vi "Spectrometer GetControlPosition.vi"(8 "error in":errorcluster, 9 "Control Refnum":refnum<vi>, 10 "Motor Name":T1=enum."Hole", 11 "Automation Refnum In":refnum<k7>) -> (0 "error out":errorcluster, 2 "Position":variant, 3 "Automation Refnum Out":refnum<k7>)   [LabVIEW 2014]
uses:
  MoveMotor Motor Name.ctl
  GetMotorPosition Mode.ctl
  Acquire Mode.ctl
panel:
  # "LICENSED MATERIALS – PROPERTY OF IBM\nCopyright IBM Corp. 2016,\nALL RIGHTS RESERVED"
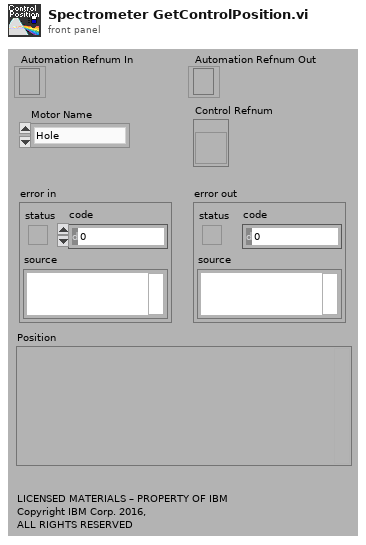
[diagram p1: front panel]
types:
  T1 = typedef "MoveMotor Motor Name.ctl" = enum16{"Spectro", "Premono", "Grating", "Slit", "Hole", "X", "Y", "XT", "YT", "XL", "YL", "Z", "Laser", "Filter", "Objective", "Detector", "Detector Temperature"}
  T2 = typedef "GetMotorPosition Mode.ctl" = u16
  T3 = typedef "Acquire Mode.ctl" = u16
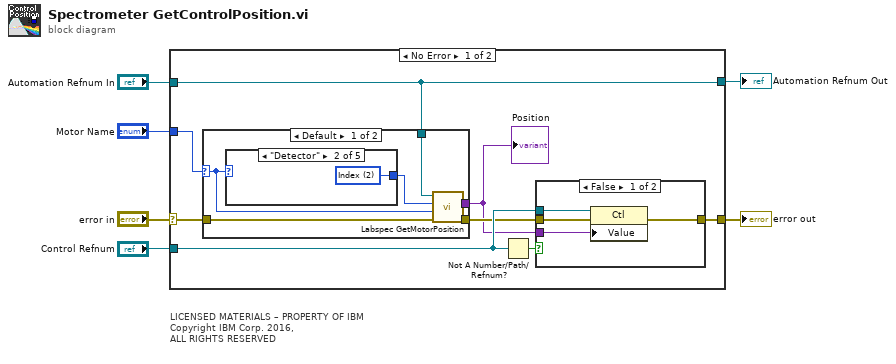
[diagram p0: block diagram]
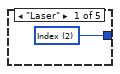
[diagram p2: hidden frame]
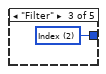
[diagram p3: hidden frame]
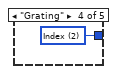
[diagram p4: hidden frame]
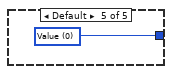
[diagram p5: hidden frame]
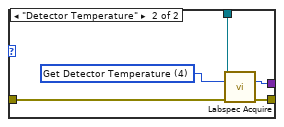
[diagram p6: hidden frame]
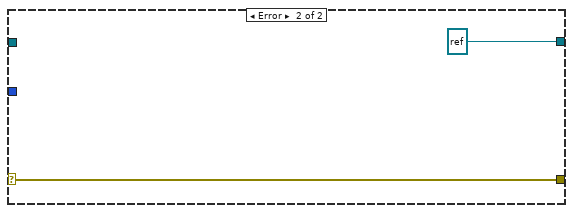
[diagram p8: hidden frame]
diagram:
  # "LICENSED MATERIALS – PROPERTY OF IBM\nCopyright IBM Corp. 2016,\nALL RIGHTS RESERVED"
  n1 = case shown="No Error" "error in" {
    selector: "error in" -> [w12 w37]
    tunnel: "Automation Refnum In" -> [w11 _]
    tunnel: [w11 refnum<k7> refnum ("Automation Refnum")] -> w5
    tunnel: "Motor Name" -> [w7 _]
    tunnel: [w13 w37] -> w3
    tunnel: "Control Refnum" -> [w14 _]
    frame No Error {
      n2 = case shown="Default" w7 {
        selector: w7 -> [w15 _]
        tunnel: w12 -> [w20 w27]
        tunnel: w11 -> [w19 w26]
        tunnel: [w18 w28] -> w10
        tunnel: [w17 w29] -> w9
        frame Default {
          n3 = case shown="\"Detector\"" w15 {
            tunnel: [w21 w22 w23 w24 w25] -> w16
            frame "Laser" {
              w21 = T2 2 items=["Value", "Step", "Index", "Size", "Full Size"] ("Mode")
            }
            frame "Detector" {
              w22 = T2 2 items=["Value", "Step", "Index", "Size", "Full Size"] ("Mode")
            }
            frame "Filter" {
              w23 = T2 2 items=["Value", "Step", "Index", "Size", "Full Size"] ("Mode")
            }
            frame "Grating" {
              w24 = T2 2 items=["Value", "Step", "Index", "Size", "Full Size"] ("Mode")
            }
            frame Default {
              w25 = T2 0 items=["Value", "Step", "Index", "Size", "Full Size"] ("Mode")
            }
          }
          n4 = call "Labspec GetMotorPosition.vi"("error in"=w20, "Motor Name"=w15, "Mode"=w16, "Automation Refnum In"=w19) -> ("error out"=w18:errorcluster, "Position"=w17:variant)  [unwired: 1 in, 5 out]
        }
        frame "Detector Temperature" {
          w30 = T3 4 items=["Spectrum", "Image", "Spectrum (Labspec Parameters)", "Spectral Image", "Get Detector Temperature", "Real Time Acquisition", "Set Photomultiplier Parameter", "Macro Spot", "Cancel Acquisition", "Set Detector"] ("Mode")
          n5 = call "Labspec Acquire.vi"("Automation Refnum In"=w26, "Mode"=w30, "error in"=w27) -> ("Acq"=w29:i32, "error out"=w28:errorcluster)  [unwired: 9 in, 2 out]
        }
      }
      "Position" <- w9
      n6 = Not A Number/Path/Refnum?(number/path/refnum=w14) -> (NaN/Path/Refnum?=w8:bool)
      n7 = case shown="False" w8 {
        tunnel: w14 -> [w34 _]
        tunnel: w10 -> [w33 w35]
        tunnel: [w32 w35] -> w13
        tunnel: w9 -> [w31 _]
        frame False {
          n8 = property class="Ctl"(reference=w34, error in=w33, "Value"=w31) -> (error out=w32:errorcluster)  [unwired: 1 out]
        }
        frame True {
        }
      }
    }
    frame Error {
    }
  }
  "error out" <- w3
  "Automation Refnum Out" <- w5
